vi "Test.vi"() -> ()   [LabVIEW 2019, in "LabSFTP.lvlib"]
doc: "<License>This software is distributed under the BSD 3-Clause License. For the full license please see license.txt or visit www.labvolution.com/license</License>"
uses:
  LabSFTP.lvlib
  Connection Info..cluster.ctl
  Private Public Key..cluster.ctl
  Password..cluster.ctl
  connect_password.vi
  connect_key.vi
panel:
  in  "Password":T1={"Password"="wxpp1275"}
  in  "Remote File Path Down":string="/home/pi/leakad/datafile.dat"
  in  "Download Local File Path":path=path "C:/Users/1/Desktop/管道泄露检测系统/download"
  in  "Remote File Path Up":string="/home/pi/leakad/"
  in  "Local File Up":path=path "C:/Users/1/Desktop/管道泄露检测系统/upload/txt.txt"
  in  "Remote Path":string="/home/pi/leakad/"
  in  "Private_Public Key":T2
  in  "Connection Type":enum16{"Password", "Private Key"}(ring)
  out "SFTP Method Response":string="SFTP connection closed\r\n"
  in  "error in (no error)":errorcluster
  out "isSftpConnected":bool
  in  "Connection Info.":T3={"Remote"="192.168.137.193", "Username"="pi", "Port (22)"=22}
  in  "SFTP Output":string="\r\n/home/pi/leakad/.\r\n/home/pi/leakad/txt.txt\r\n/home/pi/leakad/datafile.dat\r\n/home/pi/leakad/..\r\n/home/pi/leakad/ADS1256\r\n"
  # "Download File"
  # "Upload File"
  # "Get File List"
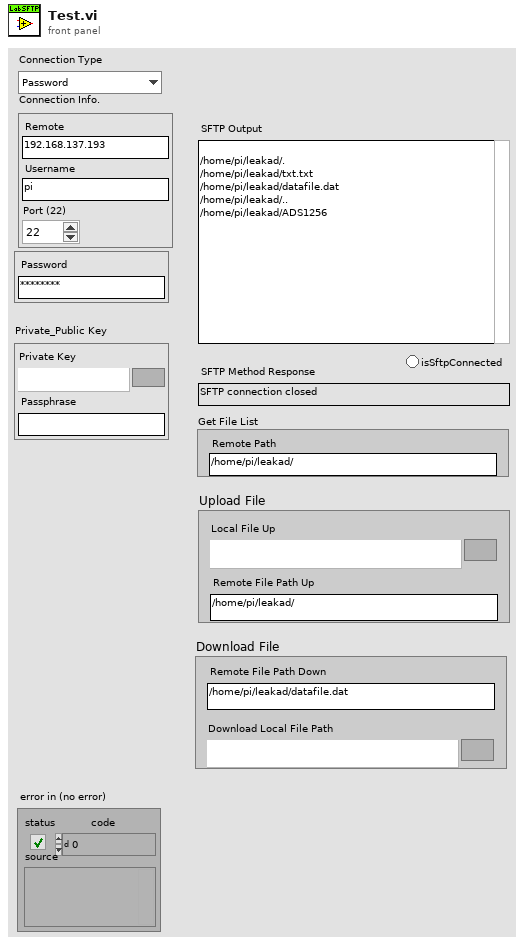
[diagram p1: front panel]
types:
  T1 = typedef "LabSFTP.lvlib/Password..cluster.ctl" = cluster{"Password":string}
  T2 = typedef "LabSFTP.lvlib/Private Public Key..cluster.ctl" = cluster{"Private Key":path, "Passphrase":string}
  T3 = typedef "LabSFTP.lvlib/Connection Info..cluster.ctl" = cluster{"Remote":string, "Username":string, "Port (22)":i32}
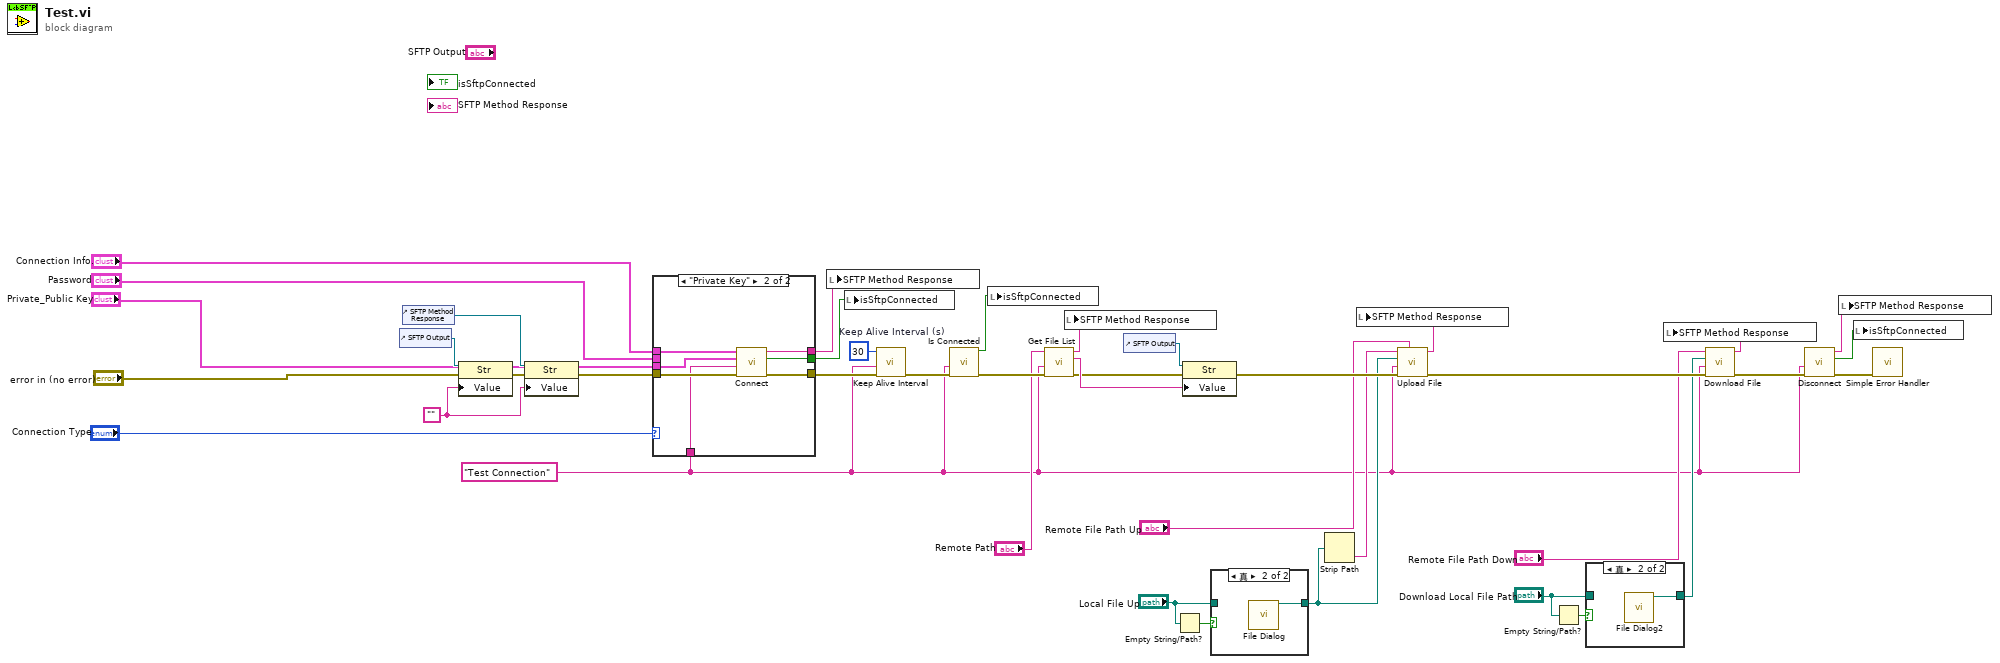
[diagram p0: block diagram]
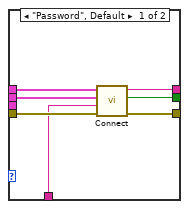
[diagram p3: hidden frame]
diagram:
  w1 = "Test Connection" ("Connection Name")
  w10 = 30  # Keep Alive Interval (s)
  w28 = ""
  n1 = control-ref of="SFTP Output"() -> (w31:refnum<vi>)
  n2 = control-ref of="SFTP Method Response"() -> (w29:refnum<vi>)
  n3 = property class="Str"(reference=w31, error in="error in (no error)", "Value"=w28) -> (error out=w32:errorcluster)  [unwired: 1 out]
  n4 = property class="Str"(reference=w29, error in=w32, "Value"=w28) -> (error out=w30:errorcluster)  [unwired: 1 out]
  n5 = case shown="\"Private Key\"" "Connection Type" {
    tunnel: [w47 w52] -> w11
    tunnel: "Connection Info." -> [w46 w54]
    tunnel: "Password" -> [w45 _]
    tunnel: [w44 w51] -> w38
    tunnel: [w43 w50] -> w36
    tunnel: w30 -> [w42 w53]
    tunnel: "Private_Public Key" -> [_ w49]
    tunnel: w1 -> [w41 w48]
    frame "Password", Default {
      n6 = call-poly "Connect.vi"("error in (no error)"=w42, "Connection Name"=w41, "Password"=w45, "Connection Info."=w46) -> ("error out"=w47:errorcluster, "isSftpConnected"=w44:bool, "Return String"=w43:string)  [unwired: 5 in]
    }
    frame "Private Key" {
      n7 = call-poly "Connect.vi"("error in (no error)"=w53, "Connection Name"=w48, "Private_Public Key"=w49, "Connection Info."=w54) -> ("error out"=w52:errorcluster, "isSshConnected"=w51:bool, "Return String"=w50:string)  [unwired: 5 in]
    }
  }
  n8 = local write "SFTP Method Response"(w36) -> ()
  n9 = local write "isSftpConnected"(w38) -> ()
  n10 = call "Keep Alive Interval.vi"("error in (no error)"=w11, "Connection Name"=w1, "Keep Alive Interval (s)"=w10) -> ("error out"=w12:errorcluster)  [unwired: 8 in]
  n11 = call "Is Connected.vi"("error in (no error)"=w12, "Connection Name"=w1) -> ("error out"=w25:errorcluster, "isSshConnected"=w37:bool)  [unwired: 8 in]
  n12 = local write "isSftpConnected"(w37) -> ()
  n13 = call "Get File List.vi"("error in (no error)"=w25, "Connection Name"=w1, "Remote Path"="Remote Path") -> ("error out"=w21:errorcluster, "File List"=w22:string, "Return String"=w24:string)  [unwired: 6 in]
  n14 = local write "SFTP Method Response"(w24) -> ()
  n15 = control-ref of="SFTP Output"() -> (w23:refnum<vi>)
  n16 = Empty String/Path?(string/path="Local File Up") -> (empty?=w9:bool)
  n17 = property class="Str"(reference=w23, error in=w21, "Value"=w22) -> (error out=w20:errorcluster)  [unwired: 1 out]
  n18 = case shown="真" w9 {
    tunnel: [w55 w56] -> w3
    tunnel: "Local File Up" -> [w55 _]
    frame False {
    }
    frame True {
      n19 = call "File Dialog"() -> ("selected path"=w56:path)  [unwired: 12 in, 3 out]
    }
  }
  n20 = Strip Path(path=w3) -> (name=w15:string)  [unwired: 1 out]
  n21 = call "Upload File.vi"("Remote Folder Path"="Remote File Path Up", "error in (no error)"=w20, "Connection Name"=w1, "Local File Path"=w3, "Remote File Name"=w15) -> ("error out"=w18:errorcluster, "Return String"=w19:string)  [unwired: 5 in]
  n22 = local write "SFTP Method Response"(w19) -> ()
  n23 = Empty String/Path?(string/path="Download Local File Path") -> (empty?=w7:bool)
  n24 = case shown="真" w7 {
    tunnel: [w57 w58] -> w4
    tunnel: "Download Local File Path" -> [w57 _]
    frame False {
    }
    frame True {
      n25 = call "File Dialog2"() -> ("selected path"=w58:path)  [unwired: 12 in, 3 out]
    }
  }
  n26 = call "Download File.vi"("error in (no error)"=w18, "Connection Name"=w1, "Local File Path"=w4, "Remote File Path"="Remote File Path Down") -> ("error out"=w17:errorcluster, "Return String"=w16:string)  [unwired: 6 in]
  n27 = local write "SFTP Method Response"(w16) -> ()
  n28 = call "Disconnect.vi"("error in (no error)"=w17, "Connection Name"=w1) -> ("error out"=w34:errorcluster, "isSshConnected"=w33:bool, "Return String"=w35:string)  [unwired: 7 in]
  n29 = local write "SFTP Method Response"(w35) -> ()
  n30 = local write "isSftpConnected"(w33) -> ()
  n31 = call <vilib>:"Simple Error Handler.vi"("error in (no error)"=w34) -> ()  [unwired: 4 in, 5 out]
